vi "SetPid&FindPos.vi"(3 "MM System":u16(ring)=1 items=["MM3000", "MM2000"]) -> (1 "Numeric":i32)   [LabVIEW 2022 SP3]
uses:
  -MotionRoutines/MotionGlobals.vi
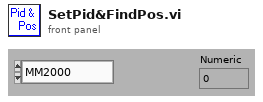
[diagram p1: front panel]
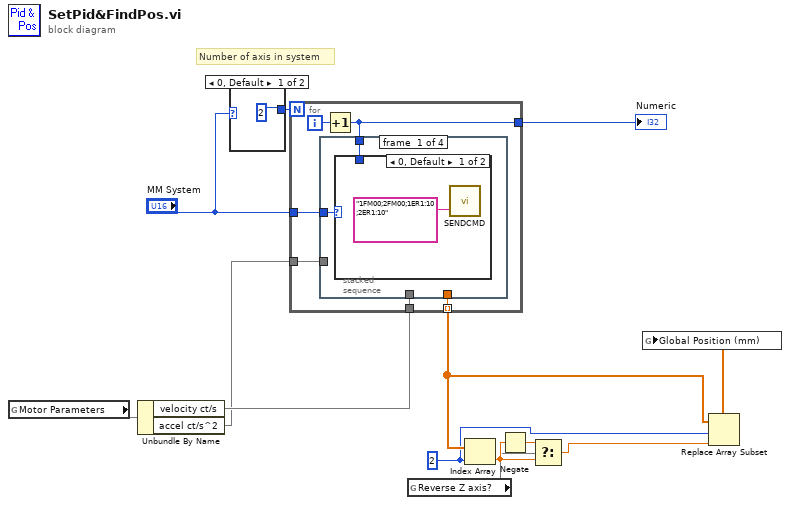
[diagram p0: block diagram]
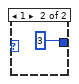
[diagram p2: hidden frame]
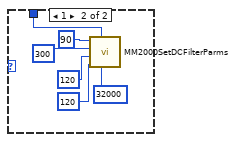
[diagram p3: hidden frame]
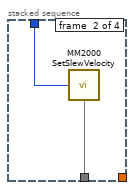
[diagram p4: hidden frame]
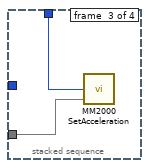
[diagram p5: hidden frame]
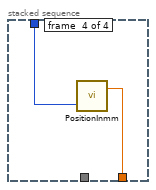
[diagram p6: hidden frame]
diagram:
  w6 = 2 ("Axis")
  # "Number of axis in system"
  n1 = global read "MotionGlobals.vi" "Motor Parameters"() -> (w3)
  n2 = Unbundle By Name(w3) -> ("velocity ct/s"=w2, "accel ct/s^2"=w1)
  n3 = case shown="0, Default" "MM System" {
    tunnel: [2 3] -> w13
    frame 0, Default {
    }
    frame 1 {
    }
  }
  n4 = for {
    N: w13 -> [_]
    tunnel: [w20] -> w8
    tunnel: [w19] -> w7 mode=indexing
    tunnel: w2 -> [w18]
    tunnel: "MM System" -> [w17]
    tunnel: w1 -> [w16]
    i -> [w21]
    n5 = Increment(x=w21) -> (x+1=w20:i32)
    n6 = stacked-sequence {
      tunnel: w20 -> [w23 w32 w34 w35]
      tunnel: [_ _ _ w36] -> w19
      tunnel: w18 -> [_ w31 _ _]
      tunnel: w17 -> [w22 _ _ _]
      tunnel: w16 -> [_ _ w33 _]
      frame #0 {
        n7 = case shown="0, Default" w22 {
          tunnel: w23 -> [_ w26]
          frame 0, Default {
            n8 = call "SENDCMD.VI"("MM2000 Command (ASCII String)"="1FM00;2FM00;1ER1:10;2ER1:10") -> ()  [unwired: 2 in, 1 out]
          }
          frame 1 {
            n9 = call "MM2000SetDCFilterParms.vi"("Following\nError (FE)"=32000 ("Following\nError (FE)"), "Axis"=w26, "Integral\nLimit (IL)"=120 ("Integral\nLimit (IL)"), "Integral\n   (KI)"=120 ("Integral\n   (KI)"), "Derivative\n      (KD)"=300 ("Derivative\n      (KD)"), "Gain\n (KP)"=90 ("Gain\n (KP)")) -> ()  [unwired: 1 in]
          }
        }
      }
      frame #1 {
        n10 = call "MM2000 SetSlewVelocity.vi"("Slew Velocity"=w31, "Axis"=w32) -> ()  [unwired: 1 in]
      }
      frame #2 {
        n11 = call "MM2000 SetAcceleration.vi"("Acceleration"=w33, "Axis"=w34) -> ()  [unwired: 1 in]
      }
      frame #3 {
        n12 = call "PositionInmm.vi"("Axis"=w35) -> ("postion in mm"=w36:dbl)  [unwired: 1 in, 1 out]
      }
    }
  }
  "Numeric" <- w8
  n13 = global read "MotionGlobals.vi" "Reverse Z axis?"() -> (w10)
  n14 = Index Array(array=w7, index=w6) -> (element=w11:dbl)
  n15 = Negate(x=w11) -> (-x=w12:dbl)
  n16 = Select(t=w12, s=w10, f=w11) -> (s? t:f=w5:dbl)
  n17 = Replace Array Subset(array=w7, new element=w5, index=w6) -> (w4:dbl[])
  n18 = global write "MotionGlobals.vi" "Global Position (mm)"(w4) -> ()
